vi "TrendPlot.vi"(10 "Y通道":string, 11 "X通道":string) -> ()   [LabVIEW 2018, in "DataDisplay.lvlib"]
uses:
  DataDisplay.lvlib
  TrendPlot/TrendPlot.lvclass
  TrendPlot/TrendPlotRef.vi
  TypeDefine/DD_DataStream.ctl
  SubVI/DD_Parameter.vi
panel:
  in  "显示时长[S]":i32=10 caption="显示时长" min=0 step=1
  in  "时长调节":bool
  in  "时间单位":enum16{"秒", "分钟", "小时"}(ring)
  in  "显示时间":bool
  in  "采样间隔[S]":dbl=10.0 caption="间隔" min=0.1 step=0.1 format="%.1f"
  in  "Y图形选择":u16(ring) items=["位移1", "位移2"]
  in  "X图形选择":u16(ring) items=["次数1", "次数2"]
  out "XY图":cluster{dbl[], dbl[]}[](graph)
  # "Y轴"
  # "秒"
  # "X轴"
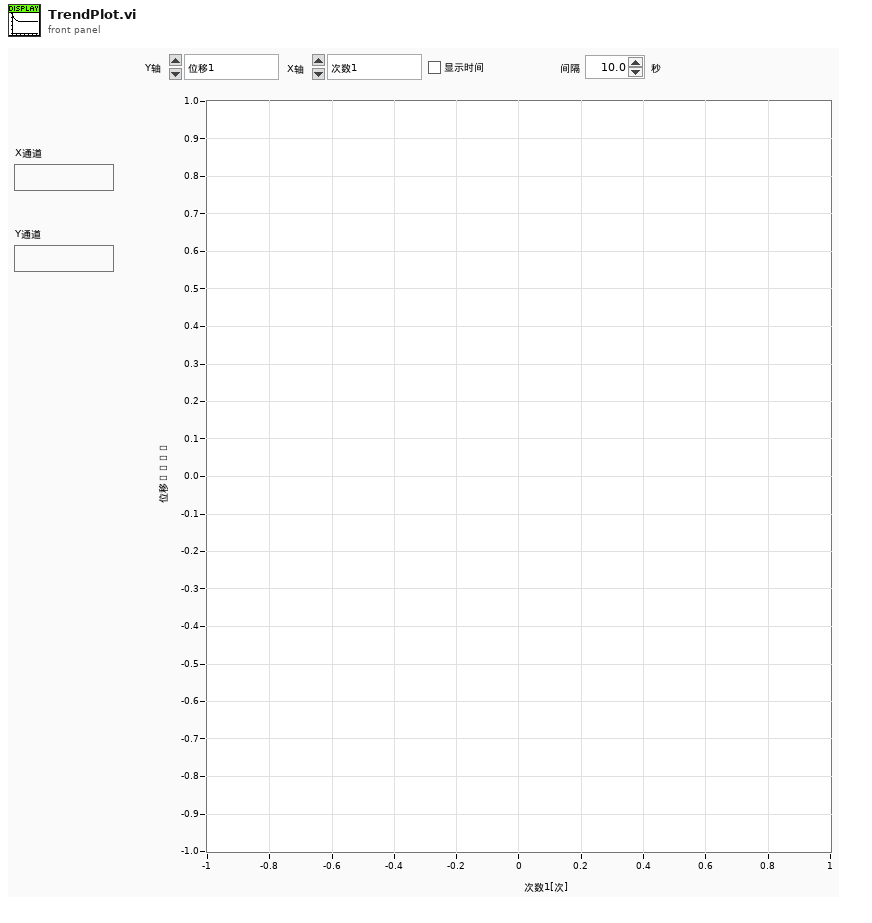
[diagram p1: front panel]
types:
  T1 = typedef "DataDisplay.lvlib/TrendPlot.lvclass/TrendPlotRef.vi" = cluster{"rVI":refnum<vi>, "rPane":refnum<vi>, "rXY图":refnum<vi>, "rX通道选择":refnum<vi>, "rY通道选择":refnum<vi>, "r采样间隔[S]":refnum<vi>, "DD_数据通知器":refnum<notifier>, "r显示时间":refnum<vi>, "r时间单位":refnum<vi>, "r时长调节":refnum<vi>, "r显示时长[S]":refnum<vi>}
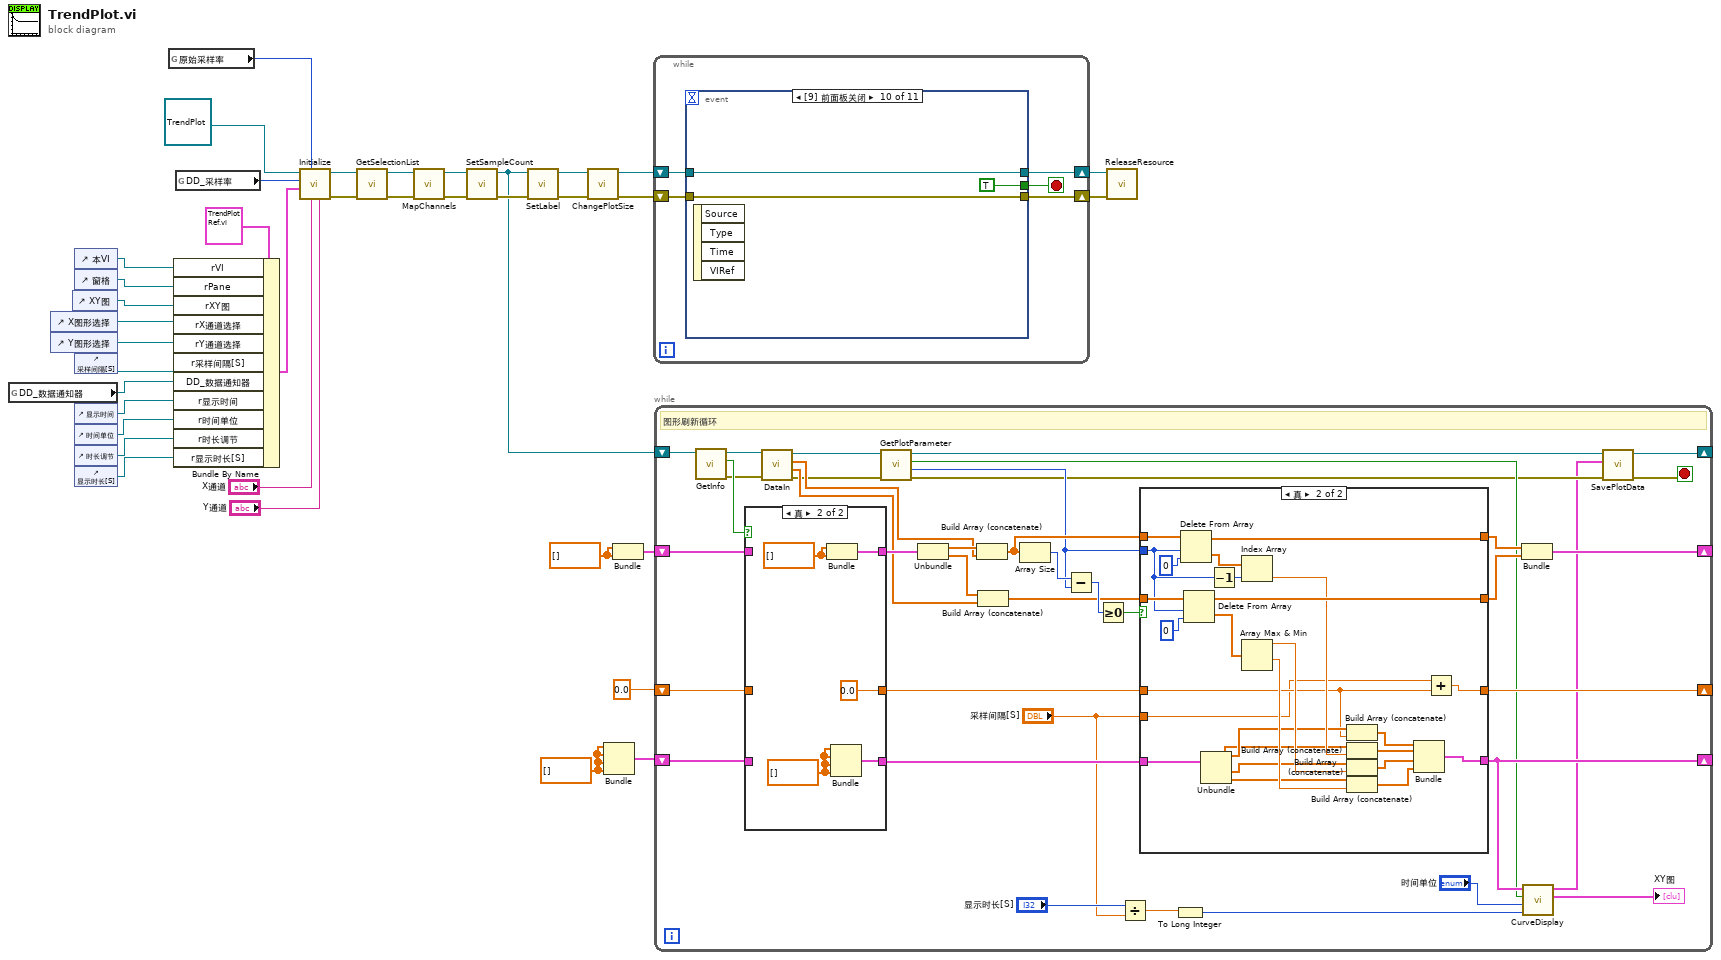
[diagram p0: block diagram]
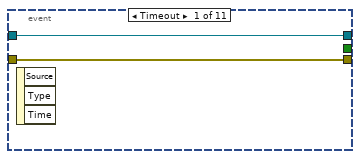
[diagram p4: hidden frame]
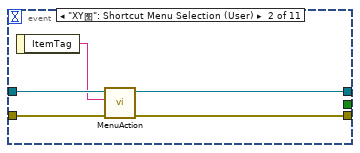
[diagram p5: hidden frame]
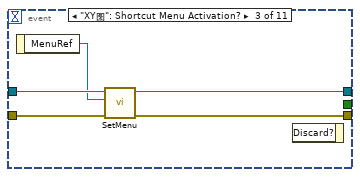
[diagram p6: hidden frame]
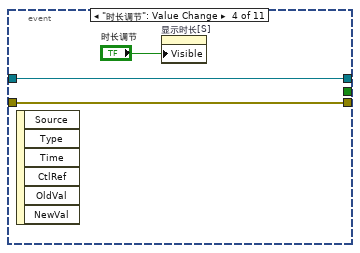
[diagram p7: hidden frame]
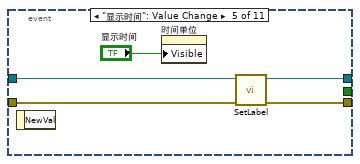
[diagram p8: hidden frame]
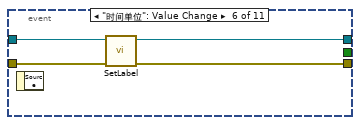
[diagram p9: hidden frame]
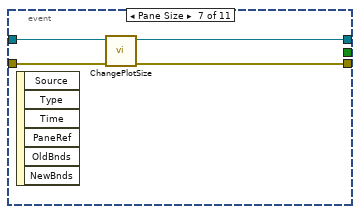
[diagram p10: hidden frame]
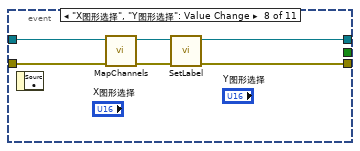
[diagram p11: hidden frame]
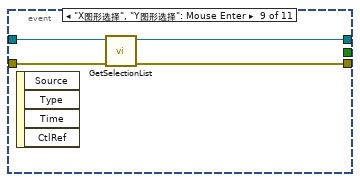
[diagram p12: hidden frame]
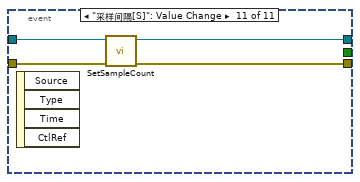
[diagram p13: hidden frame]
diagram:
  w8 = dbl[] []
  w14 = dbl[] []
  n1 = global read "DD_Parameter.vi" "DD_数据通知器"() -> (w36:refnum<notifier>)
  n2 = control-ref of="X图形选择"() -> (w33:refnum<vi>)
  n3 = control-ref of="Y图形选择"() -> (w34:refnum<vi>)
  n4 = control-ref of="XY图"() -> (w32:refnum<vi>)
  n5 = control-ref of="本VI"() -> (w30:refnum<vi>)
  n6 = control-ref of="窗格"() -> (w31:refnum<vi>)
  n7 = control-ref of="采样间隔[S]"() -> (w35:refnum<vi>)
  n8 = control-ref of="显示时间"() -> (w6:refnum<vi>)
  n9 = control-ref of="时间单位"() -> (w5:refnum<vi>)
  n10 = control-ref of="时长调节"() -> (w4:refnum<vi>)
  n11 = control-ref of="显示时长[S]"() -> (w3:refnum<vi>)
  n12 = global read "DD_Parameter.vi" "原始采样率"() -> (w17:i32)
  n13 = Bundle By Name(cluster=T1 {"rVI"=refnum, "rPane"=refnum, "rXY图"=refnum, "rX通道选择"=refnum, "rY通道选择"=refnum, "r采样间隔[S]"=refnum, "DD_数据通知器"=refnum, "r显示时间"=refnum, "r时间单位"=refnum, "r时长调节"=refnum, "r显示时长[S]"=refnum} ("引用"), "rVI"=w30, "rPane"=w31, "rXY图"=w32, "rX通道选择"=w33, "rY通道选择"=w34, "r采样间隔[S]"=w35, "DD_数据通知器"=w36, "r显示时间"=w6, "r时间单位"=w5, "r时长调节"=w4, "r显示时长[S]"=w3) -> (w29:T1)
  n14 = global read "DD_Parameter.vi" "DD_采样率"() -> (w37:i32)
  n15 = call "Initialize.vi"("Y通道"="Y通道", "X通道"="X通道", "原始采样率[Hz]"=w17, "引用"=w29, "显示采样率[Hz]"=w37, "XYPlot 输入"=refnum<class "TrendPlot.lvclass"> refnum ("DataDisplay.lvlib:TrendPlot.lvclass")) -> ("error out"=w27:errorcluster, "XYPlot 输出"=w18:refnum<class "TrendPlot.lvclass">)  [unwired: 4 in]
  n16 = call "GetSelectionList.vi"("error in (no error)"=w27, "XYPlot 输入"=w18) -> ("error out"=w26:errorcluster, "XYPlot 输出"=w28:refnum<class "TrendPlot.lvclass">)  [unwired: 8 in]
  n17 = call "MapChannels.vi"("error in (no error)"=w26, "XYPlot 输入"=w28) -> ("error out"=w25:errorcluster, "XYPlot 输出"=w11:refnum<class "TrendPlot.lvclass">)  [unwired: 8 in]
  n18 = call "SetSampleCount.vi"("error in (no error)"=w25, "XYPlot 输入"=w11) -> ("error out"=w12:errorcluster, "XYPlot 输出"=w10:refnum<class "TrendPlot.lvclass">)  [unwired: 8 in]
  n19 = call "SetLabel.vi"("error in (no error)"=w12, "XYPlot 输入"=w10) -> ("error out"=w20:errorcluster, "XYPlot 输出"=w22:refnum<class "TrendPlot.lvclass">)  [unwired: 8 in]
  n20 = call "ChangePlotSize.vi"("error in (no error)"=w20, "XYPlot 输入"=w22) -> ("error out"=w19:errorcluster, "XYPlot 输出"=w21:refnum<class "TrendPlot.lvclass">)  [unwired: 8 in]
  n21 = Bundle(w8, w8, w8, w8) -> (w9:cluster{dbl[], dbl[], dbl[], dbl[]})  [unwired: 1 in]
  n22 = Bundle(w14, w14) -> (w13:cluster{dbl[], dbl[]})  [unwired: 1 in]
  n23 = while {
    shift-right: [w39] -> w24
    shift-left: w21 -> [w41]
    shift-right: [w38] -> w23
    shift-left: w19 -> [w40]
    stop <- w42 stop-if-true
    n24 = event shown="[9] 前面板关闭" {
      selector: _ -> [_ _ _ _ _ _ _ _ _ _ _]
      dyn-events: _ -> [_ _ _ _ _ _ _ _ _ _ _]
      timeout: _ -> [_ _ _ _ _ _ _ _ _ _ _]
      tunnel: [_ _ _ _ _ _ _ _ _ TRUE _] -> w42
      tunnel: w41 -> [w44 w47 w52 w57 w60 w64 w70 w76 w80 w82 w85]
      tunnel: w40 -> [w43 w49 w54 w56 w62 w66 w69 w73 w79 w81 w87]
      tunnel: [w44 w46 w51 w57 w59 w63 w67 w74 w78 w82 w84] -> w39
      tunnel: [w43 w48 w53 w56 w61 w65 w68 w71 w77 w81 w86] -> w38
      event Timeout {
        n25 = event-data() -> ()  [unwired: 1 in, 3 out]
      }
      event "XY图": Shortcut Menu Selection (User) {
        n26 = event-data() -> ("ItemTag"=w45:string)  [unwired: 1 in]
        n27 = call "MenuAction.vi"("error in (no error)"=w49, "项标识符"=w45, "TrendPlot 输入"=w47) -> ("error out"=w48:errorcluster, "TrendPlot 输出"=w46:refnum<class "TrendPlot.lvclass">)  [unwired: 7 in]
      }
      event "XY图": Shortcut Menu Activation? {
        n28 = event-data() -> ("MenuRef"=w50:refnum<k9>)  [unwired: 1 in]
        n29 = call "SetMenu.vi"("error in (no error)"=w54, "菜单引用"=w50, "TrendPlot 输入"=w52) -> ("error out"=w53:errorcluster, "TrendPlot 输出"=w51:refnum<class "TrendPlot.lvclass">)  [unwired: 7 in]
        n30 = event-data() -> ()  [unwired: 2 in, 1 out]
      }
      event "时长调节": Value Change {
        n31 = event-data() -> ()  [unwired: 1 in, 6 out]
        n32 = property on="显示时长[S]" class="DigNum (严格)"("Visible"="时长调节") -> ()  [unwired: 2 in, 2 out]
      }
      event "显示时间": Value Change {
        n33 = event-data() -> ()  [unwired: 1 in, 1 out]
        n34 = property on="时间单位" class="Enum (严格)"("Visible"="显示时间") -> ()  [unwired: 2 in, 2 out]
        n35 = call "SetLabel.vi"("error in (no error)"=w62, "XYPlot 输入"=w60) -> ("error out"=w61:errorcluster, "XYPlot 输出"=w59:refnum<class "TrendPlot.lvclass">)  [unwired: 8 in]
      }
      event "时间单位": Value Change {
        n36 = event-data() -> ()  [unwired: 1 in, 1 out]
        n37 = call "SetLabel.vi"("error in (no error)"=w66, "XYPlot 输入"=w64) -> ("error out"=w65:errorcluster, "XYPlot 输出"=w63:refnum<class "TrendPlot.lvclass">)  [unwired: 8 in]
      }
      event Pane Size {
        n38 = event-data() -> ()  [unwired: 1 in, 6 out]
        n39 = call "ChangePlotSize.vi"("error in (no error)"=w69, "XYPlot 输入"=w70) -> ("error out"=w68:errorcluster, "XYPlot 输出"=w67:refnum<class "TrendPlot.lvclass">)  [unwired: 8 in]
      }
      event "X图形选择", "Y图形选择": Value Change {
        n40 = event-data() -> ()  [unwired: 1 in, 1 out]
        n41 = call "MapChannels.vi"("error in (no error)"=w73, "XYPlot 输入"=w76) -> ("error out"=w72:errorcluster, "XYPlot 输出"=w75:refnum<class "TrendPlot.lvclass">)  [unwired: 8 in]
        n42 = call "SetLabel.vi"("error in (no error)"=w72, "XYPlot 输入"=w75) -> ("error out"=w71:errorcluster, "XYPlot 输出"=w74:refnum<class "TrendPlot.lvclass">)  [unwired: 8 in]
      }
      event "X图形选择", "Y图形选择": Mouse Enter {
        n43 = event-data() -> ()  [unwired: 1 in, 4 out]
        n44 = call "GetSelectionList.vi"("error in (no error)"=w79, "XYPlot 输入"=w80) -> ("error out"=w77:errorcluster, "XYPlot 输出"=w78:refnum<class "TrendPlot.lvclass">)  [unwired: 8 in]
      }
      event Panel Close {
        n45 = event-data() -> ()  [unwired: 1 in, 4 out]
      }
      event "采样间隔[S]": Value Change {
        n46 = event-data() -> ()  [unwired: 1 in, 4 out]
        n47 = call "SetSampleCount.vi"("error in (no error)"=w87, "XYPlot 输入"=w85) -> ("error out"=w86:errorcluster, "XYPlot 输出"=w84:refnum<class "TrendPlot.lvclass">)  [unwired: 8 in]
      }
    }
  }
  n48 = while {
    shift-right: [w105] -> _
    shift-left: w13 -> [w118]
    shift-right: [w92] -> _
    shift-left: w10 -> [w121]
    shift-right: [w99] -> _
    shift-left: w9 -> [w104]
    shift-right: [w100] -> _
    shift-left: 0.0 -> [w101]
    stop <- w91 stop-if-true
    # "图形刷新循环"
    n49 = call "GetInfo.vi"("XYPlot 输入"=w121) -> ("error out"=w114:errorcluster, "通道变更"=w116:bool, "XYPlot 输出"=w115:refnum<class "TrendPlot.lvclass">)  [unwired: 8 in]
    n50 = case shown="真" w116 {
      tunnel: w118 -> [w129 _]
      tunnel: [w129 w133] -> w117
      tunnel: w104 -> [w128 _]
      tunnel: [w128 w132] -> w103
      tunnel: [w127 0.0] -> w102
      tunnel: w101 -> [w127 _]
      frame False {
      }
      frame True {
        w131 = dbl[] []
        w134 = dbl[] []
        n51 = Bundle(w134, w134) -> (w133:cluster{dbl[], dbl[]})  [unwired: 1 in]
        n52 = Bundle(w131, w131, w131, w131) -> (w132:cluster{dbl[], dbl[], dbl[], dbl[]})  [unwired: 1 in]
      }
    }
    n53 = call "DataIn.vi"("error in (no error)"=w114, "XYPlot 输入"=w115) -> ("error out"=w110:errorcluster, "Data1"=w112:dbl[], "Data0"=w113:dbl[], "XYPlot 输出"=w111:refnum<class "TrendPlot.lvclass">)  [unwired: 6 in]
    n54 = call "GetPlotParameter.vi"("error in (no error)"=w110, "XYPlot 输入"=w111) -> ("error out"=w90:errorcluster, "采样点数"=w108:i32, "时间轴"=w98:bool, "XYPlot 输出"=w109:refnum<class "TrendPlot.lvclass">)  [unwired: 6 in]
    n55 = Unbundle(w117) -> (w120:dbl[], w119:dbl[])
    n56 = Build Array (concatenate)(w120, w113) -> (w126:dbl[])
    n57 = Build Array (concatenate)(w119, w112) -> (w122:dbl[])
    n58 = Array Size(array=w126) -> (size(s)=w125:i32)
    n59 = Subtract(x=w125, y=w108) -> (x-y=w123:i32)
    n60 = Greater Or Equal To 0?(x=w123) -> (x >= 0?=w124:bool)
    n61 = Divide(x="显示时长[S]", y="采样间隔[S]") -> (x/y=w94:dbl)
    n62 = case shown="真" w124 {
      tunnel: w126 -> [w138 w164]
      tunnel: [w138 w161] -> w107
      tunnel: w122 -> [w137 w162]
      tunnel: [w137 w159] -> w106
      tunnel: w108 -> [_ w156]
      tunnel: w103 -> [w136 w154]
      tunnel: [w136 w150] -> w99
      tunnel: w102 -> [w135 w145]
      tunnel: [w135 w144] -> w100
      tunnel: "采样间隔[S]" -> [_ w139]
      frame False {
      }
      frame True {
        n63 = Delete From Array(array=w164, length=w156, index=0 ("索引")) -> (deleted portion=w157:dbl[], array with subset deleted=w161:dbl[])
        n64 = Delete From Array(array=w162, length=w156, index=0 ("索引")) -> (deleted portion=w158:dbl[], array with subset deleted=w159:dbl[])
        n65 = Unbundle(w154) -> (w149:dbl[], w148:dbl[], w147:dbl[], w146:dbl[])
        n66 = Decrement(x=w156) -> (x-1=w155:i32)
        n67 = Index Array(array=w157, index=w155) -> (element=w153:dbl)
        n68 = Array Max & Min(array=w158) -> (max value=w152:dbl, min value=w151:dbl)  [unwired: 2 out]
        n69 = Build Array (concatenate)(w149, w145) -> (w143:dbl[])
        n70 = Build Array (concatenate)(w148, w153) -> (w142:dbl[])
        n71 = Build Array (concatenate)(w147, w152) -> (w141:dbl[])
        n72 = Build Array (concatenate)(w146, w151) -> (w140:dbl[])
        n73 = Bundle(w143, w142, w141, w140) -> (w150:cluster{dbl[], dbl[], dbl[], dbl[]})  [unwired: 1 in]
        n74 = Add(x=w139, y=w145) -> (x+y=w144:dbl)
      }
    }
    n75 = To Long Integer(number=w94) -> (32bit integer=w93:i32)
    n76 = Bundle(w107, w106) -> (w105:cluster{dbl[], dbl[]})  [unwired: 1 in]
    n77 = call "CurveDisplay.vi"("曲线点数"=w93, "时间单位"="时间单位", "时间显示"=w98, "数据"=w99) -> ("图形输出"=→"XY图":cluster{"数组":dbl[], "数组":dbl[]}[], "数据输出"=w88:cluster{"数组":dbl[]}[])  [unwired: 6 in]
    n78 = call "SavePlotData.vi"("error in (no error)"=w90, "数据输入"=w88, "TrendPlot 输入"=w109) -> ("error out"=w91:errorcluster, "TrendPlot 输出"=w92:refnum<class "TrendPlot.lvclass">)  [unwired: 7 in]
  }
  n79 = call "ReleaseResource.vi"("error in (no error)"=w23, "XYPlot 输入"=w24) -> ()  [unwired: 8 in, 2 out]
